vi "WP Vector on GIC 3.vi"(1 "GIC Output 2":T1={"Real/Sim"=FALSE, "WP Lats and Longs"={"WP Lats"=[], "WP Longs"=[]}, "GPS Time Int"=0.0, "GPS Com Port"="", "Compass Com Port"="", "Prop Com Port"="", "GPS Data"=[], "Compass"=0.0, "LMS Vector"=[], "Vision Vector"=[], "Direction Cmd"=0.0, "Speed Cmd"=0.0, "Time of Last GPS"=0.0, "WP Vector"=[], "WP Number"=0, "Num of WPs"=0, "SW Map"=[], "Obst Lats and Longs"={"Obst Lats"=[], "Obst Longs"=[]}, "Parameters"=[], "Path Cluster"={"Path x nodes"=[], "Path y nodes"=[]}, "     Use ?\nOff       On"=[TRUE, TRUE, FALSE, FALSE]} {"Obst Lats and Longs"."Obst Longs" format="%#_8g"; "Obst Lats and Longs"."Obst Lats" format="%#_8g"}) -> (0 "GIC Output":T1={"Real/Sim"=FALSE, "WP Lats and Longs"={"WP Lats"=[], "WP Longs"=[]}, "GPS Time Int"=0.0, "GPS Com Port"="", "Compass Com Port"="", "Prop Com Port"="", "GPS Data"=[], "Compass"=0.0, "LMS Vector"=[], "Vision Vector"=[], "Direction Cmd"=0.0, "Speed Cmd"=0.0, "Time of Last GPS"=0.0, "WP Vector"=[], "WP Number"=0, "Num of WPs"=0, "SW Map"=[], "Obst Lats and Longs"={"Obst Lats"=[], "Obst Longs"=[]}, "Parameters"=[], "Path Cluster"={"Path x nodes"=[], "Path y nodes"=[]}, "     Use ?\nOff       On"=[TRUE, TRUE, FALSE, FALSE]} {"Obst Lats and Longs"."Obst Longs" format="%#_8g"; "Obst Lats and Longs"."Obst Lats" format="%#_8g"})   [LabVIEW 2014]
panel:
  # "GPS"
  # "LMS"
  # "Vision"
  # "Prop"
  # "GPS"
  # "LMS"
  # "Vision"
  # "Prop"
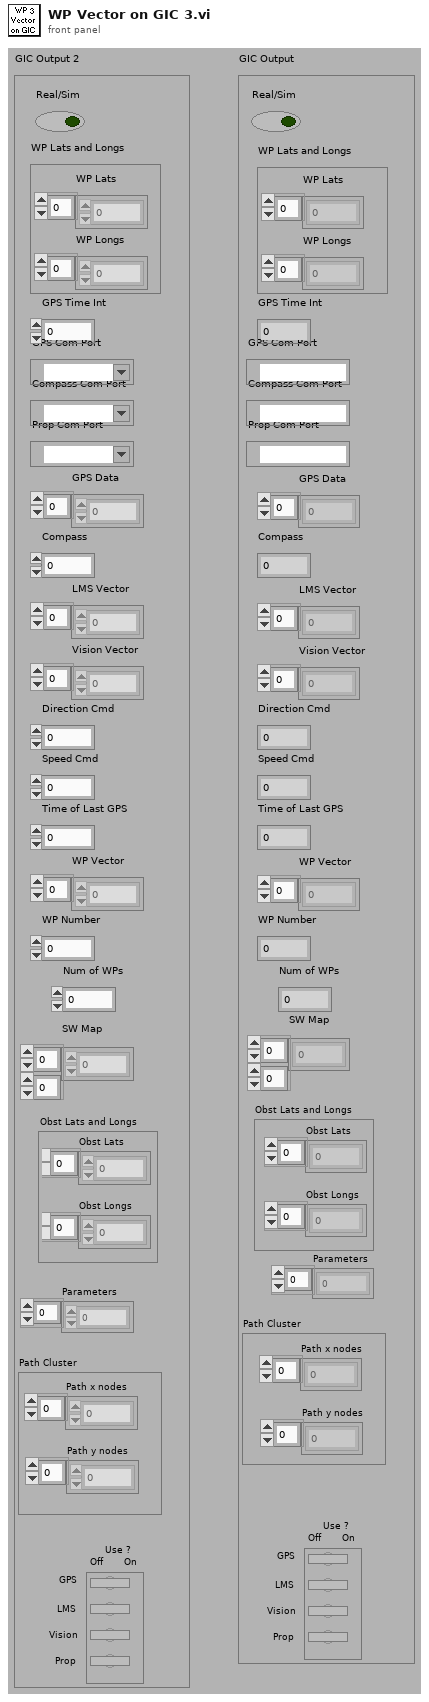
[diagram p1: front panel]
types:
  T1 = cluster{"Real/Sim":bool, "WP Lats and Longs":cluster{"WP Lats":dbl[], "WP Longs":dbl[]}, "GPS Time Int":dbl, "GPS Com Port":refnum<visa-resource-name>, "Compass Com Port":refnum<visa-resource-name>, "Prop Com Port":refnum<visa-resource-name>, "GPS Data":dbl[], "Compass":dbl, "LMS Vector":dbl[], "Vision Vector":dbl[], "Direction Cmd":dbl, "Speed Cmd":dbl, "Time of Last GPS":dbl, "WP Vector":dbl[], "WP Number":i32, "Num of WPs":i16, "SW Map":i32[][], "Obst Lats and Longs":cluster{"Obst Lats":dbl[], "Obst Longs":dbl[]}, "Parameters":dbl[], "Path Cluster":cluster{"Path x nodes":dbl[], "Path y nodes":dbl[]}, "     Use ?\nOff       On":bool[]}
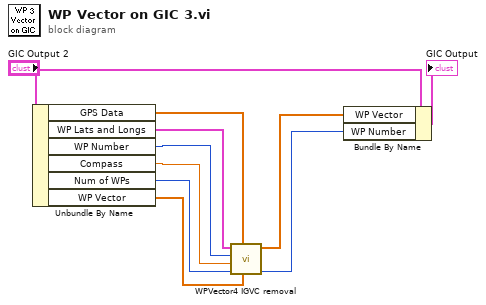
[diagram p0: block diagram]
diagram:
  n1 = Unbundle By Name("GIC Output 2") -> ("GPS Data"=w6:dbl[], "WP Lats and Longs"=w5:cluster{"WP Lats":dbl[], "WP Longs":dbl[]}, "WP Number"=w4:i32, "Compass"=w3:dbl, "Num of WPs"=w2:i16, "WP Vector"=w1:dbl[])
  n2 = call "WPVector4 IGVC removal.vi"("WP Vector Input"=w1, "Robot Lat and Long"=w6, "Num of WPs"=w2, "Heading"=w3, "WP Num Input"=w4, "All WPs Cluster"=w5) -> ("WP Number"=w10:i32, "Angle in degrees and Distance in meters"=w9:dbl[])  [unwired: 4 in]
  n3 = Bundle By Name(cluster="GIC Output 2", "WP Vector"=w9, "WP Number"=w10) -> (→"GIC Output":T1)
